vi "3ph Power from 9239 (TESTER).vi"() -> ()   [LabVIEW 2019]
doc: "Demonstrates how to implement basic power measurement on a three-phase electrical power system, such as power and energy values, frequency amplitudes, and symmetrical components."
uses:
  Instruments and Measurement IO/PTs and CTs/3ph Inputs.ctl
  <vilib>/DAQmx/read.llb/DAQmx Read (Analog 1D Wfm NChan NSamp).vi
  <vilib>/DAQmx/create/channels.llb/DAQmx Create Channel (AI-Voltage-Basic).vi
  <vilib>/DAQmx/configure/timing.llb/DAQmx Timing (Sample Clock).vi
  <vilib>/DAQmx/miscellaneous.llb/DAQmx Fill In Error Info.vi
  <vilib>/addons/Electrical Power/Basic/Measurement/Frequency (N Channels).vi
  <vilib>/addons/Electrical Power/Basic/Measurement/RMS (N Channels).vi
  <vilib>/addons/Electrical Power/Basic/Measurement/Power (N Channels).vi
  <vilib>/addons/Electrical Power/Basic/Measurement/Energy (N Channels).vi
  <vilib>/addons/Electrical Power/Basic/NI_EP_Basic.lvlib
  <resource>/objmgr/daqmx.rc
panel:
  in  "3 Phase Current Scaling":dbl[](array[numeric])=[-12.724, -12.739, -12.73]
  in  "3 Phase Voltage Scaling":dbl[](array[numeric])=[50.0, 50.0, 50.0]
  in  "?":bool
  out "Power Array":dbl[](array[numeric])
  out "Current 2":waveform(dbl)[](graph)
  out "Voltages 2":waveform(dbl)[](graph)
  out "SampClk.Rate":dbl
  out "Iteration":i32
  in  "3ph Inputs":T1={"voltage channels"="Mod3/ai0:2, Mod4/ai0:2", "minimum voltage value"=-10.0, "maximum voltage value"=10.0, "3ph sample rate [Hz]"=5000.0, "3phf samples per channel"=500, "Voltage Scaling"=100.0, "Current Scaling"=100.0} {"Current Scaling" format="%0.2f"; "Voltage Scaling" format="%0.2f"; "3phf samples per channel" format="%0.2f"; "3ph sample rate [Hz]" format="%0.2f"; "maximum voltage value" format="%0.2f"; "minimum voltage value" format="%0.2f"}
  out "error out":errorcluster
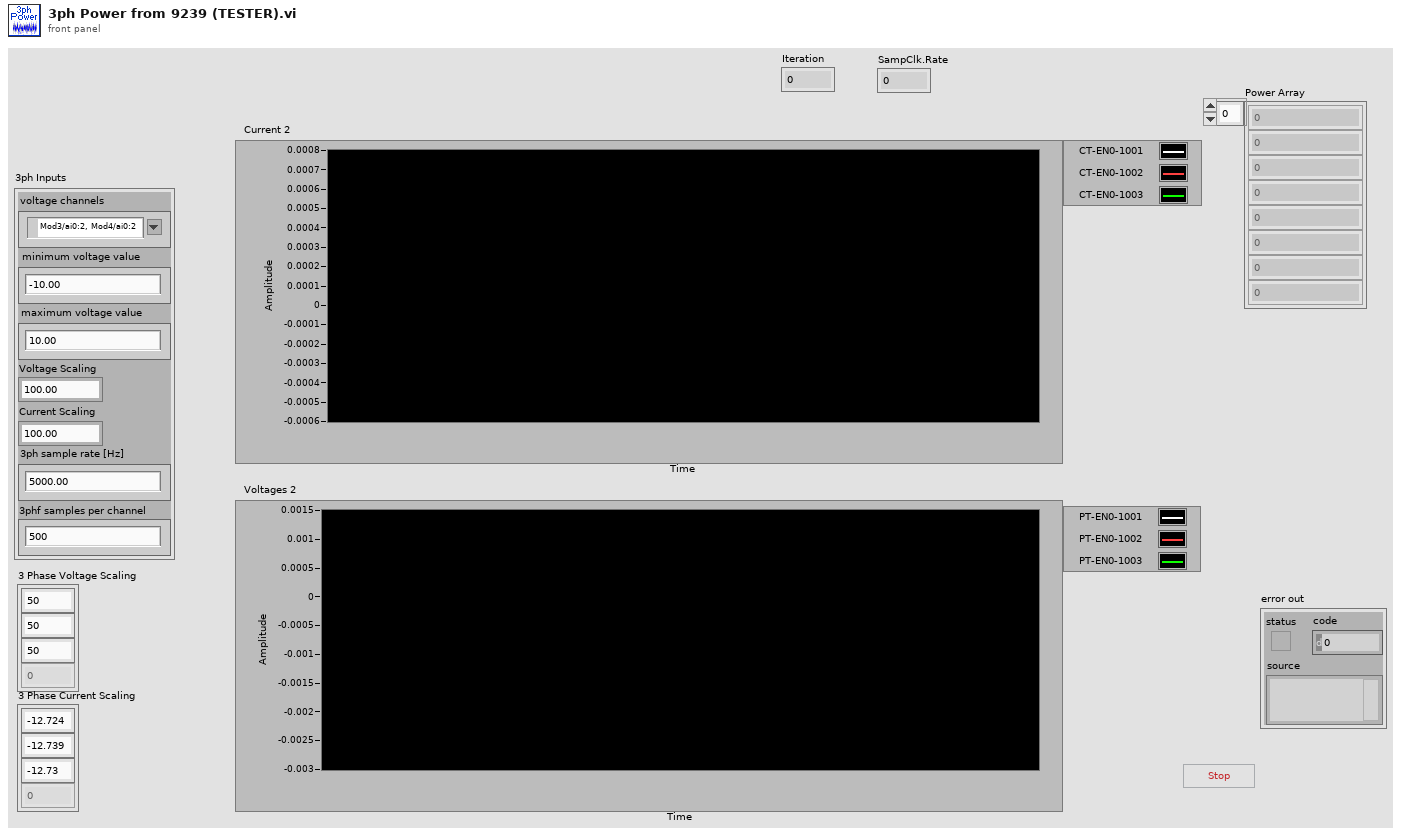
[diagram p1: front panel]
types:
  T1 = typedef "3ph Inputs.ctl" = cluster{"voltage channels":tag, "minimum voltage value":dbl, "maximum voltage value":dbl, "3ph sample rate [Hz]":dbl, "3phf samples per channel":i32, "Voltage Scaling":dbl, "Current Scaling":dbl}
  T2 = typedef "NI_EP_Basic.lvlib/basic_Power Value.ctl" = cluster{"active power [W]":dbl, "apparent power [VA]":dbl, "reactive power [VAR]":dbl, "power factor":dbl}
  T3 = typedef "NI_EP_Basic.lvlib/basic_Energy Value.ctl" = cluster{"active energy [Wh]":dbl, "apparent energy [VAh]":dbl, "reactive energy [VARh]":dbl}
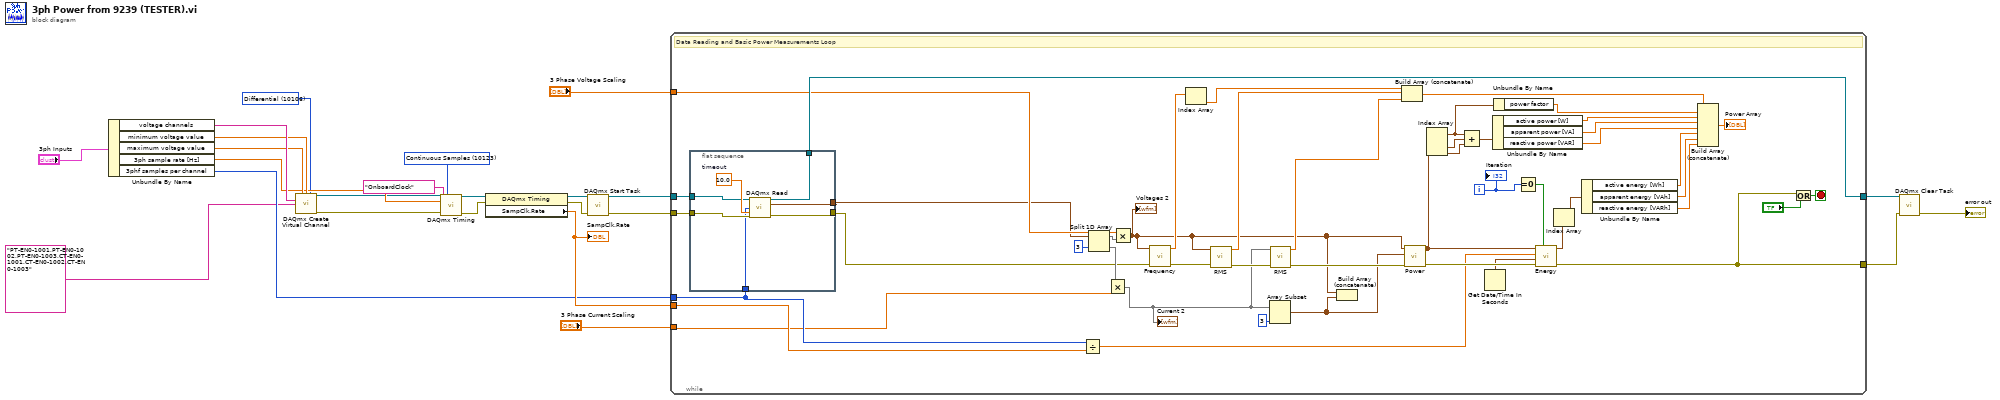
[diagram p0: block diagram]
diagram:
  w7 = 10106 items=["Default"=-1, "RSE"=10083, "NRSE"=10078, "Differential"=10106, "Pseudodifferential"=12529] ("input terminal configuration")
  w22 = 10123 items=["Finite Samples"=10178, "Continuous Samples"=10123] ("sample mode")
  n1 = Unbundle By Name("3ph Inputs") -> ("voltage channels"=w14:tag, "minimum voltage value"=w13:dbl, "maximum voltage value"=w12:dbl, "3ph sample rate [Hz]"=w11:dbl, "3phf samples per channel"=w10:i32)
  n2 = call-poly <vilib>:"DAQmx Create Virtual Channel.vi"("maximum value"=w12, "minimum value"=w13, "input terminal configuration"=w7, "physical channels"=w14, "name to assign"="PT-EN0-1001,PT-EN0-1002,PT-EN0-1003,CT-EN0-1001,CT-EN0-1002,CT-EN0-1003") -> ("task out"=w9:refnum<k21>, "error out"=w8:errorcluster)  [unwired: 9 in]
  n3 = call-poly <vilib>:"DAQmx Timing.vi"("task/channels in"=w9, "sample mode"=w22, "rate"=w11, "source"=tag "OnboardClock", "error in"=w8) -> ("task out"=w20:refnum<k21>, "error out"=w18:errorcluster)  [unwired: 9 in]
  n4 = property class="DAQmx Timing"(reference=w20, error in=w18) -> (reference out=w19:refnum<k21>, error out=w17:errorcluster, "SampClk.Rate"=w16:dbl)
  "SampClk.Rate" <- w16
  n5 = call <vilib>:"DAQmx Start Task.vi"("task/channels in"=w19, "error in"=w17) -> ("task out"=w24:refnum<k21>, "error out"=w21:errorcluster)  [unwired: 12 in]
  n6 = while {
    tunnel: w24 -> [w31]
    tunnel: [w69] -> w23
    tunnel: w16 -> [w38]
    tunnel: w10 -> [w37]
    tunnel: [w32] -> w3
    tunnel: "3 Phase Voltage Scaling" -> [w28]
    tunnel: "3 Phase Current Scaling" -> [w33]
    tunnel: w21 -> [w70]
    i -> [w36]
    stop <- w71 stop-if-true
    # "Data Reading and Basic Power Measurements Loop"
    n7 = flat-sequence {
      tunnel: w70 -> [w78]
      tunnel: [w77] -> w69
      tunnel: [w72] -> w25
      tunnel: [w75] -> w39
      tunnel: w37 -> [w74]
      tunnel: w31 -> [w73]
      frame #0 {
        w76 = 10.0  # timeout
        n8 = call-poly <vilib>:"DAQmx Read.vi"("task/channels in"=w73, "number of samples per channel"=w74, "timeout"=w76, "error in"=w78) -> ("task out"=w77:refnum<k21>, "data"=w72:waveform(dbl)[], "error out"=w75:errorcluster)  [unwired: 9 in]
      }
    }
    n9 = Divide(x=w37, y=w38) -> (x/y=w63:dbl)
    n10 = Split 1D Array(array=w25, index=3) -> (first subarray=w58:waveform(dbl)[], second subarray=w57:waveform(dbl)[])
    n11 = Multiply(x=w57, y=w33) -> (x*y=w29:waveform(dbl)[])
    "Current 2" <- w29
    n12 = Multiply(x=w28, y=w58) -> (x*y=w30:waveform(dbl)[])
    "Voltages 2" <- w30
    n13 = call-poly <vilib>:"Frequency.vi"("error in (no error)"=w39, "waveforms"=w30) -> ("error out"=w68:errorcluster, "frequencies"=w67:dbl[])  [unwired: 8 in]
    n14 = Index Array(array=w67) -> (element=w52:dbl)  [unwired: 1 in]
    n15 = call-poly <vilib>:"RMS.vi"("error in (no error)"=w68, "waveforms"=w30) -> ("error out"=w61:errorcluster, "RMS values"=w35:dbl[])  [unwired: 8 in]
    n16 = Array Subset(array=w29, length=3) -> (w56:waveform(dbl)[])  [unwired: 1 in]
    n17 = call-poly <vilib>:"RMS.vi"("error in (no error)"=w61, "waveforms"=w29) -> ("error out"=w60:errorcluster, "RMS values"=w34:dbl[])  [unwired: 8 in]
    n18 = Build Array (concatenate)(w30, w56) -> ()  [unwired: 1 out]
    n19 = Build Array (concatenate)(w52, w35, w34) -> (w51:dbl[])
    n20 = call-poly <vilib>:"Power.vi"("error in (no error)"=w60, "current waveforms"=w56, "voltage waveforms"=w30) -> ("error out"=w66:errorcluster, "power values"=w55:T2[])  [unwired: 7 in]
    n21 = Index Array(array=w55) -> (element #1=w44:T2, element #2=w47:T2, element #3=w46:T2)  [unwired: 3 in]
    n22 = Compound Arithmetic op=ADD(w44, w47, w46) -> (w45:T2)
    n23 = Get Date/Time In Seconds() -> (seconds since 1Jan1904=w65:timestamp)
    n24 = Unbundle By Name(w45) -> ("active power [W]"=w40:dbl, "apparent power [VA]"=w42:dbl, "reactive power [VAR]"=w41:dbl)
    n25 = Unbundle By Name(w44) -> ("power factor"=w43:dbl)
    n26 = Equal To 0?(x=w36) -> (x = 0?=w64:bool)
    n27 = call-poly <vilib>:"Energy.vi"("reset? (F)"=w64, "error in (no error)"=w66, "start timestamp"=w65, "interval length [s]"=w63, "power values"=w55) -> ("error out"=w32:errorcluster, "energy values"=w54:T3[])  [unwired: 4 in, 1 out]
    n28 = Index Array(array=w54) -> (element=w53:T3)  [unwired: 1 in]
    n29 = Unbundle By Name(w53) -> ("active energy [Wh]"=w50:dbl, "apparent energy [VAh]"=w49:dbl, "reactive energy [VARh]"=w48:dbl)
    n30 = Build Array (concatenate)(w51, w43, w40, w42, w41, w50, w49, w48) -> (→"Power Array":dbl[])
    n31 = Or(x=w32, y="?") -> (x .or. y?=w71:bool)
    "Iteration" <- w36
  }
  n32 = call <vilib>:"DAQmx Clear Task.vi"("task in"=w23, "error in"=w3) -> ("error out"=→"error out":errorcluster)  [unwired: 13 in]
